vi "test VIT Verify Scripting Code.VITester.vi"(8 "error in":errorcluster, 11 "Testing Approval Tests in":refnum<class "VITester Extension Tests.lvclass">) -> (0 "error out":errorcluster, 3 "Testing Approval Tests out":refnum<class "VITester Extension Tests.lvclass">)   [LabVIEW 2026, in "VITester Extension Tests.lvclass"]
uses:
  VITester Extension Tests.lvclass
  VITester Extension Tests.lvclass/VITester Extension Tests.ctl
  Source/Extensions/VITester.Extension/VITester.Extension.lvlib
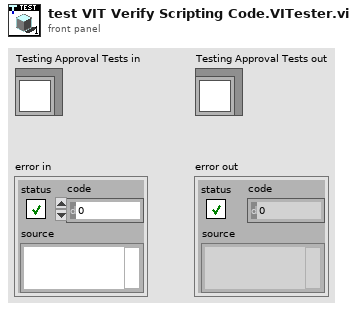
[diagram p1: front panel]
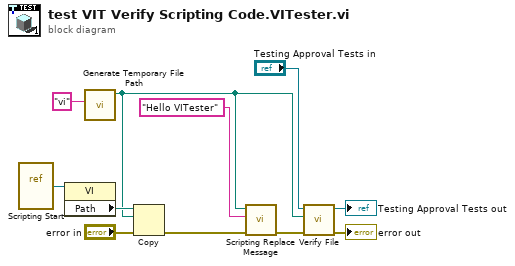
[diagram p0: block diagram]
diagram:
  n1 = vi-ref "Scripting Start.vi"() -> (w6:refnum<vi>)
  n2 = property on="Property Node" class="VI"(reference=w6) -> ("Path"=w4:path)  [unwired: 1 in, 2 out]
  n3 = call <vilib>:"Generate Temporary File Path.vi"("Temporary File Extension (tmp)"="vi") -> ("Unique Temporary File Path"=w2:path)  [unwired: 9 in, 1 out]
  n4 = Copy(8:"error in", 10:w2, 11:w4) -> (0:w1:errorcluster)  [unwired: 2 in, 2 out]
  n5 = call "Scripting Replace Message.vi"("error in"=w1, "New Message"="Hello VITester", "Path"=w2) -> ("error out"=w9:errorcluster)  [unwired: 8 in]
  n6 = call "Verify File.vi"("error in"=w9, "Path to Binary File to Verify"=w2, "TestCase in"="Testing Approval Tests in") -> ("error out"=→"error out":errorcluster, "TestCase out"=→"Testing Approval Tests out":refnum<class "VITester Extension Tests.lvclass">)  [unwired: 7 in]
